vi "PH_DIM.add String Service.vi"(0 "i ref in":refnum<vi>, 1 "Service Name":string="N/A", 2 "String":string, 3 "String Length (1024)":u16=1024, 5 "error in (no error)":errorcluster) -> (14 "i ref out":refnum<vi>, 17 "Service ID":i32, 19 "error out":errorcluster)   [LabVIEW 2014, in "PH_Common.lvlib"]
doc: "This VI opens a string service \"<instancename>_ServiceName\", if no error comes in, the string size is not 0 and the Service Name is not N/A. For further use, the Service ID is given out (it is \"-1\" if the service has not been added)."
uses:
  PH_Common.lvlib
  lib.lib/UtilityLib/UtilityLib.lvlib
  lib.lib/DimLVEvent/LVDimInterface/LVDimInterface.lvlib
  CSCore/CSSystem/CSSystemLib/CSSystemLib.lvlib
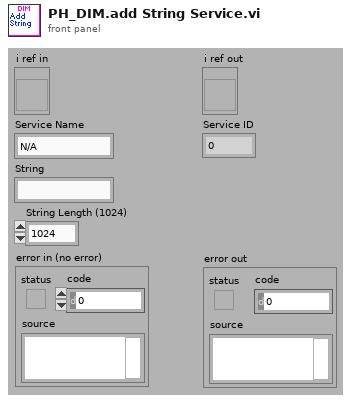
[diagram p1: front panel]
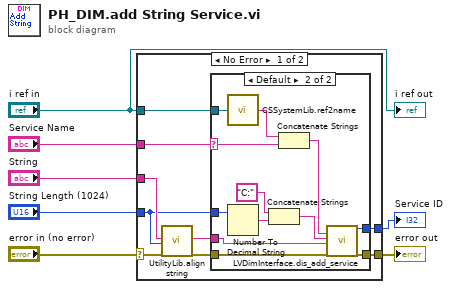
[diagram p0: block diagram]
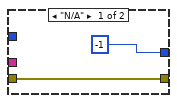
[diagram p2: hidden frame]
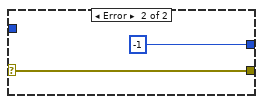
[diagram p3: hidden frame]
diagram:
  n1 = case shown="No Error" "error in (no error)" {
    selector: "error in (no error)" -> [w8 w32]
    tunnel: [w16 -1 ("my_serviceID")] -> w7
    tunnel: [w15 w32] -> w6
    tunnel: "String" -> [w14 _]
    tunnel: "i ref in" -> [w13 _]
    tunnel: "Service Name" -> [w12 _]
    tunnel: "String Length (1024)" -> [w9 _]
    frame No Error {
      n2 = call "UtilityLib.align string.vi"("stringIn"=w14, "stringLength (80)"=w9, "error in (no error)"=w8) -> ("stringOut"=w11:string, "error out"=w10:errorcluster)  [unwired: 15 in]
      n3 = case shown="Default" w12 {
        selector: w12 -> [_ w24]
        tunnel: [-1 ("my_serviceID") w30] -> w16
        tunnel: [w18 w29] -> w15
        tunnel: w13 -> [_ w26]
        tunnel: w10 -> [w18 w25]
        tunnel: w11 -> [_ w23]
        tunnel: w9 -> [_ w19]
        frame "N/A" {
        }
        frame Default {
          n4 = call "CSSystemLib.ref2name.vi"("obj refnum"=w26) -> ("name"=w27:string)
          n5 = Number To Decimal String(number=w19) -> (decimal integer string=w20:string)  [unwired: 1 in]
          n6 = Concatenate Strings("C:" ("typeDescriptor"), w20) -> (w21:string)
          n7 = Concatenate Strings(w27, w24) -> (w28:string)
          n8 = call "LVDimInterface.dis_add_service.vi"("serviceName"=w28, "typeDescriptor"=w21, "data"=w23, "error in (no error)"=w25) -> ("my_serviceID"=w30:i32, "error out"=w29:errorcluster)  [unwired: 14 in]
        }
      }
    }
    frame Error {
    }
  }
  "Service ID" <- w7
  "error out" <- w6
  "i ref out" <- "i ref in"
